vi "get unique id.vi"(11 "identifying queue in":refnum<class "identifying queue.lvclass">) -> (3 "unique id":string)   [LabVIEW 2015, in "identifying queue.lvclass"]
uses:
  identifying queue.lvclass
  identifying queue.lvclass/identifying queue.ctl
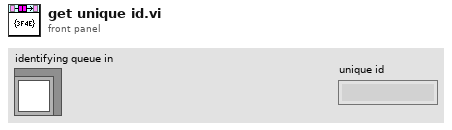
[diagram p1: front panel]
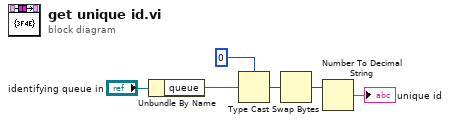
[diagram p0: block diagram]
diagram:
  n1 = Unbundle By Name("identifying queue in") -> ("queue"=w5:refnum<queue>)
  n2 = Type Cast(type=u64 0, x=w5) -> (*(type *) &x=w2:u64)
  n3 = Swap Bytes(anything=w2) -> (byte swapped=w1:u64)
  n4 = Number To Decimal String(number=w1) -> (decimal integer string=→"unique id":string)  [unwired: 1 in]
